vi "Get Required Driver Type.vi"(8 "error in (no error)":errorcluster, 11 "Instrument Msg in":refnum<class "Instrument Msg.lvclass">) -> (0 "error out":errorcluster, 2 "Required Driver Type":refnum<class "Instrument Driver.lvclass">, 3 "Instrument Msg out":refnum<class "Instrument Msg.lvclass">)   [LabVIEW 2020, in "Instrument Handler.lvlib" / "Instrument Msg.lvclass"]
doc: "Get the Required Driver Type for execution of the Instrument Msg."
uses:
  Instrument Msg.lvclass
  PPL/HDH.Actor Framework.Core.Instrument Driver.lvlibp/Instrument Driver/Instrument Driver.lvclass
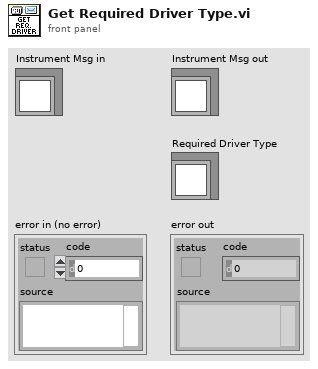
[diagram p1: front panel]
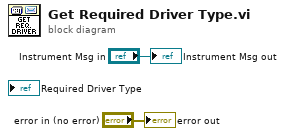
[diagram p0: block diagram]
diagram:
  "error out" <- "error in (no error)"
  "Instrument Msg out" <- "Instrument Msg in"
